vi "Cannon Fix.vi"(1 "Cannon Info Modified":T2, 2 "Cannon Info Original":T2) -> (0 "Cannon Info Fixed":T2)   [LabVIEW 2013]
uses:
  <vilib>/Rock Robotics/WPI/Relay/WPI_RelayValue.ctl
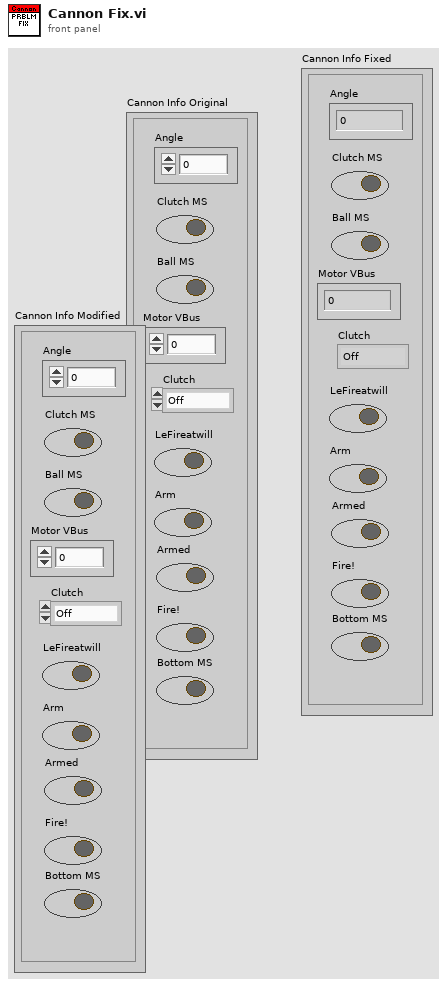
[diagram p1: front panel]
types:
  T1 = typedef "WPI_RelayValue.ctl" = enum16{"Off", "On", "Forward", "Reverse"}
  T2 = cluster{"Angle":dbl, "Clutch MS":bool, "Ball MS":bool, "Clutch ":T1, "LeFireatwill":bool, "Arm":bool, "Armed":bool, "Fire!":bool, "Bottom MS":bool, "Motor VBus":dbl}
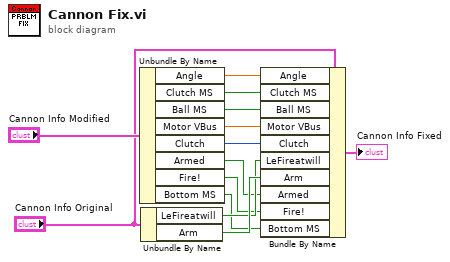
[diagram p0: block diagram]
diagram:
  n1 = Unbundle By Name("Cannon Info Modified") -> ("Angle"=w9:dbl, "Clutch MS"=w8:bool, "Ball MS"=w7:bool, "Motor VBus"=w10:dbl, "Clutch"=w11:T1, "Armed"=w6:bool, "Fire!"=w5:bool, "Bottom MS"=w4:bool)
  n2 = Unbundle By Name("Cannon Info Original") -> ("LeFireatwill"=w12:bool, "Arm"=w13:bool)
  n3 = Bundle By Name(cluster="Cannon Info Original", "Angle"=w9, "Clutch MS"=w8, "Ball MS"=w7, "Motor VBus"=w10, "Clutch"=w11, "LeFireatwill"=w12, "Arm"=w13, "Armed"=w6, "Fire!"=w5, "Bottom MS"=w4) -> (→"Cannon Info Fixed":T2)
